vi "LIDAR V5.1 Mem1 Manager.vi"(6 "SignalMem":refnum<k21>="SignalMem", 7 "FIFO IN":refnum<k21>="AI FIFOO", 10 "FIFO Out":refnum<k21>="Out FIFOO", 11 "Source Clk":refnum<k21>="130MHz") -> ()   [LabVIEW 2015]
uses:
  <vilib>/Platform/TimedLoop/XDataNode/timing_clust.ctl
  <vilib>/Platform/TimedLoop/XDataNode/nitl_modes.ctl
  <vilib>/Platform/TimedLoop/XDataNode/wakeup.ctl
  <vilib>/rvi/Emulation/niFpgaSctlEmulationGetInTimedLoop.vi
  <vilib>/rvi/Emulation/niFpgaEmulationReportErrorSimple.vi
  <vilib>/rvi/Emulation/niFpgaGetClockAttributes.vi
  <vilib>/rvi/Emulation/niFpgaCriticalErrorInLSC.vi
  <vilib>/rvi/DataTransferAndStorage/Container/Common/niFpgaContainerExecOnDevCompGetState.vi
  <vilib>/rvi/Emulation/niFpgaEmulationIsFPGAContextNoSignature.vi
  <vilib>/rvi/DataTransferAndStorage/Container/Common/niFpgaContainerGetUniqueNameForEmu.vi
  <vilib>/rvi/Emulation/niFpgaProcessEmulError.vi
  <vilib>/rvi/errors/nirviReportUnexpectedCaseInternalError (U32).vi
  <vilib>/rvi/Memory/Memory_Emulation/niFpgaMemoryEmulationCacheClearOnFirstRun.vi
  <vilib>/rvi/Memory/Memory_Emulation/nirvimemoryEmulationManagerCache_MakeExclusive.vi
  <vilib>/rvi/Memory/Memory_Emulation/niFpgaMemoryEmulationValidateCache.vi
  <vilib>/rvi/Memory/Memory_Emulation/nirvimemoryEmulationManagerCache_InsertValue.vi
  <vilib>/Utility/error.llb/Clear Errors.vi
  <vilib>/rvi/Memory/Memory_Emulation/nirvimemoryEmulationManagerCache_ReleaseExclusive.vi
  <vilib>/rvi/Memory/Memory_Emulation/nirvimemoryEmulationManagerCache_GetValue.vi
  <vilib>/rvi/Memory/Memory_Emulation/nirvimemoryEmulationManagerCache_SetValue.vi
  <vilib>/rvi/Emulation/niFpgaSctlEmulationResourceMgr.vi
  <vilib>/rvi/errors/niFpgaSetErrorForExecOnDevCompSimple.vi
  <vilib>/rvi/eio/common/nirviEmuReportErrorAndStop.vi
  <vilib>/rvi/FIFO/Fifo_Resource/nirvififoEmulationSetSize.vi
  <vilib>/rvi/FIFO/Fifo_Resource/nirviFifoEmulationQueueMgr.vi
  <instcachedir>/0/nirviFifoEmulationQueueMgr_E5CAEC123FF24DC58D834DCA3CDAA9B5.lvgen/nirviFifoEmulationQueueMgr_E5CAEC123FF24DC58D834DCA3CDAA9B5_001.vi
  <vilib>/rvi/FIFO/Fifo_Resource/nirvififoEmulationDetermineInputValidOut.vi
  <vilib>/rvi/FIFO/Fifo_Resource/nirvififoEmulationCreateLock.vi
  <vilib>/rvi/FIFO/Fifo_Resource/nirvififoEmulationObtainLock.vi
  <vilib>/rvi/FIFO/Fifo_Resource/nirvififoEmulationReleaseLock.vi
  <vilib>/rvi/occurrence/nirviWaitOnOccurrenceBase.vi
  <vilib>/rvi/errors/nirviReportUnexpectedCaseInternalError.vi
  <vilib>/rvi/interface/RandomDataEmulation/niFpgaRandomDataHandleErrors.vi
  <vilib>/Platform/TimedLoop/XDataNode/XDataNode.xnode
  <vilib>/rvi/FXPMathLib/FxpAdd/XNode/nifxpmath_Add.xnode
  <vilib>/rvi/DataTransferAndStorage/Container/XNode/niFpgaContainer.xnode
  <vilib>/rvi/Memory/Memory_Emulation/niFpgaMemoryEmulationRefIn.vi
  <vilib>/rvi/FIFO/Fifo_Resource/niFpgaFifoEmulationRefIn.vi
  <vilib>/Platform/TimedLoop/XDataNode/XDNodeRunTimeDep.lvlib
  <vilib>/rvi/FXPMathLib/sim/FxpSim.dll
panel:
  in  "Mode":bool
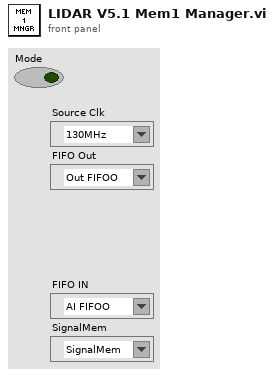
[diagram p1: front panel]
types:
  T1 = typedef "XDNodeRunTimeDep.lvlib/timing_clust.ctl" = cluster{"Expected End [f-1]":u64, "Actual End [f-1]":u64, "Finished Late? [f-1]":bool, "Expected End [i-1]":u64, "Actual End [i-1]":u64, "Finished Late? [i-1]":bool, "Expected Start [i]":u64, "Actual Start [i]":u64, "Expected Start [f]":u64, "Actual Start [f]":u64, "Source Name":string, "Structure Name":string, "Period":i64, "Deadline":i64, "Offset":i64, "Start":i64, "Priority":i32, "Timeout":i32, "Mode":T2, "Wakeup Reason":T3, "Error":errorcluster, "Source Type":string, "Secondary Source Type":string, "Global End Time":u64, "Global Start Time":u64, "Frame Duration":u64, "Iteration Duration":u64, "Assigned CPU":i32, "I/O Scan Engine Mode":u32}
  T2 = typedef "XDNodeRunTimeDep.lvlib/nitl_modes.ctl" = enum32{"No Change", "Process missed periods, maintain original phase", "Discard missed periods, maintain original phase", "Process missed periods, ignore original phase", "Discard missed periods, ignore original phase"}
  T3 = typedef "XDNodeRunTimeDep.lvlib/wakeup.ctl" = enum32{"Normal", "Aborted", "Asynchronous wakeup", "Timing source error", "Timed loop error", "Timeout"}
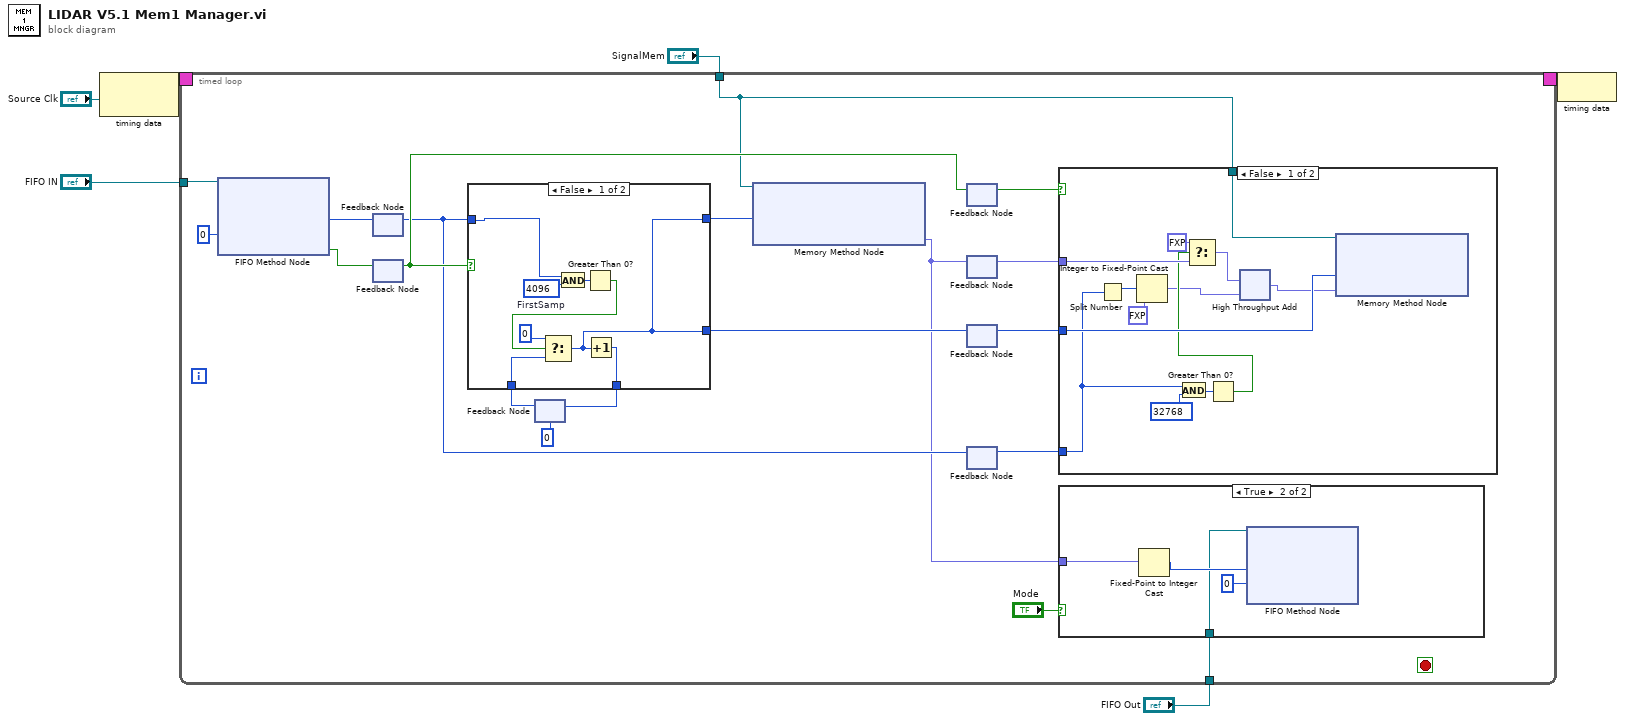
[diagram p0: block diagram]
diagram:
  n1 = node-c288("Source Clk") -> (w6:T1)
  n2 = timed-loop {
    timing: w6 -> [_]
    timing-out: [_] -> w5
    tunnel: "FIFO IN" -> [w21]
    tunnel: "SignalMem" -> [w20]
    tunnel: "FIFO Out" -> [w10]
    stop <- _ stop-if-true
    n3 = xnode ("FIFO Method Node")("Timeout"=0, "FIFO In"=w21) -> ("Element"=w25:u32, "Timed Out?"=w23:bool)  [unwired: 1 out]
    n4 = feedback-in #1(w25) -> ()
    n5 = feedback #1() -> (w9:u32)  [unwired: 1 in]
    n6 = feedback-in #2(w23) -> ()
    n7 = feedback #2() -> (w22:bool)  [unwired: 1 in]
    n8 = feedback #3(u32 0 ("Element")) -> (w11:u32)
    n9 = case shown="False" w22 {
      tunnel: w9 -> [w49 _]
      tunnel: [w43 _] -> w14
      tunnel: [w44 w51] -> w12
      tunnel: w11 -> [w45 w51]
      tunnel: [w43 w51] -> w19
      frame False {
        w50 = u32 4096  # FirstSamp
        n10 = And(x=w49, y=w50) -> (x .and. y?=w48:u32)
        n11 = Greater Than 0?(x=w48) -> (x > 0?=w47:bool)
        n12 = Select(t=u32 0 ("Element"), s=w47, f=w45) -> (s? t:f=w43:u32)
        n13 = Increment(x=w43) -> (x+1=w44:u32)
      }
      frame True {
      }
    }
    n14 = feedback-in #3(w12) -> ()
    n15 = xnode ("Memory Method Node")("Address"=w14, "Memory In"=w20) -> ("Data"=w7:fxp<+/-,22,22>)  [unwired: 1 out]
    n16 = feedback-in #4(w22) -> ()
    n17 = feedback #4() -> (w18:bool)  [unwired: 1 in]
    n18 = feedback-in #5(w7) -> ()
    n19 = feedback #5() -> (w17:fxp<+/-,22,22>)  [unwired: 1 in]
    n20 = feedback-in #6(w19) -> ()
    n21 = feedback #6() -> (w16:u32)  [unwired: 1 in]
    n22 = feedback-in #7(w9) -> ()
    n23 = feedback #7() -> (w15:u32)  [unwired: 1 in]
    n24 = case shown="False" w18 {
      tunnel: w17 -> [w41 _]
      tunnel: w15 -> [w31 _]
      tunnel: w16 -> [w39 _]
      tunnel: w20 -> [w37 _]
      frame False {
        n25 = Split Number(x=w31) -> (hi(x)=w32:u16)  [unwired: 1 out]
        n26 = Integer to Fixed-Point Cast(fixed-point type=fxp<+/-,16,16> 0.0, integer=w32) -> (fixed-point=w30:fxp<+/-,16,16>)
        n27 = And(x=w31, y=u32 32768) -> (x .and. y?=w35:u32)
        n28 = Greater Than 0?(x=w35) -> (x > 0?=w34:bool)
        n29 = Select(t=fxp<+/-,22,22> 0.0, s=w34, f=w41) -> (s? t:f=w40:fxp<+/-,22,22>)
        n30 = xnode ("High Throughput Add")("x"=w40, "y"=w30) -> ("x+y"=w38:fxp<+/-,22,22>)
        n31 = xnode ("Memory Method Node")("Address"=w39, "Data"=w38, "Memory In"=w37) -> ()  [unwired: 1 out]
      }
      frame True {
      }
    }
    n32 = case shown="True" "Mode" {
      tunnel: w10 -> [_ w26]
      tunnel: w7 -> [_ w28]
      frame False {
      }
      frame True {
        n33 = Fixed-Point to Integer Cast(1:w28) -> (0:w27:i32)
        n34 = xnode ("FIFO Method Node")("Element"=w27, "Timeout"=0, "FIFO In"=w26) -> ()  [unwired: 2 out]
      }
    }
  }
  n35 = node-c288(w5) -> ()
